vi "2-2.vi"() -> ()   [LabVIEW 2019, in "2.lvlib"]
uses:
  2.lvlib
  <vilib>/Utility/file.llb/Read Delimited Spreadsheet (string).vi
panel:
  out "XY Graph":cluster{i32[], i32[]}(graph)
  out "aim":i32
  out "depth x distance":i32
  out "distance":i32
  out "depth":i32
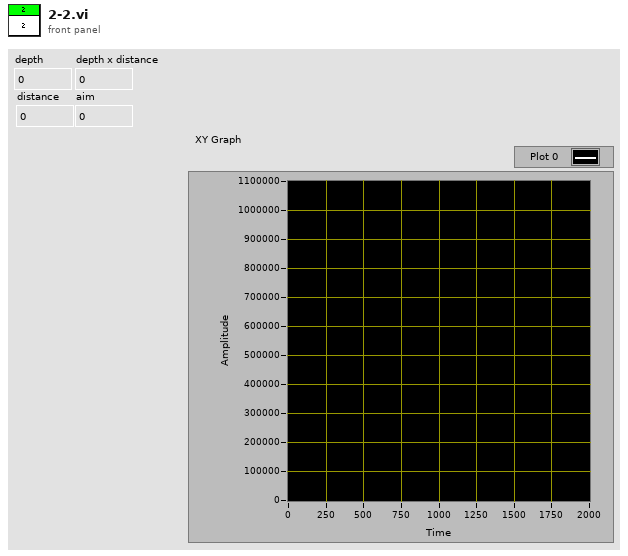
[diagram p1: front panel]
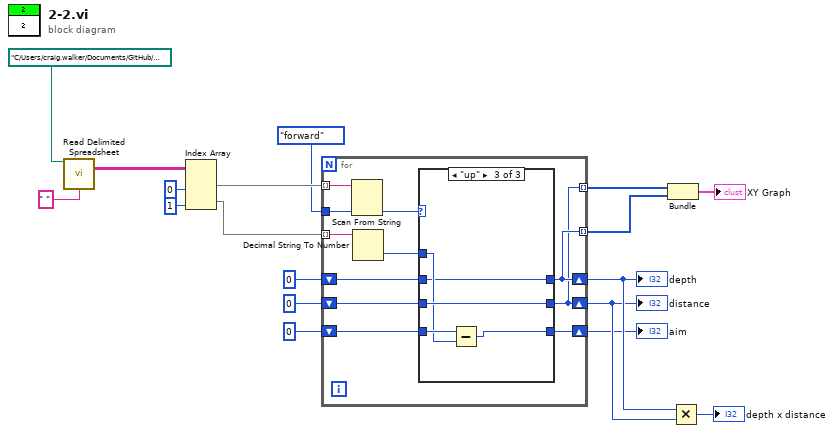
[diagram p0: block diagram]
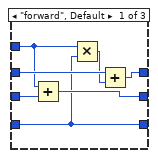
[diagram p2: hidden frame]
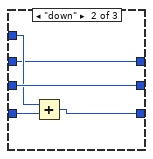
[diagram p3: hidden frame]
diagram:
  n1 = call-poly <vilib>:"Read Delimited Spreadsheet.vi"("file path (dialog if empty)"=path "C:/Users/craig.walker/Documents/GitHub/lv2019-Advent-of-Code-2021/2/input.txt", "delimiter (\\t)"=" " ("delimiter (\\t)")) -> ("all rows"=w1:string[][])  [unwired: 8 in, 5 out]
  n2 = Index Array(array=w1, index (col) #1=0 ("disabled index (col)"), index (col) #2=1 ("index (col)")) -> (element #1=w16:string[], element #2=w12:string[])  [unwired: 2 in]
  n3 = for {
    tunnel: w16 -> [w29] mode=indexing
    tunnel: enum16{"forward", "down", "up"}."forward" -> [w28]
    tunnel: w12 -> [w27] mode=indexing
    shift-right: [w20] -> w9
    shift-left: 0 -> [w25]
    shift-right: [w19] -> w8
    shift-left: 0 -> [w23]
    shift-right: [w21] -> w5
    shift-left: 0 -> [w22]
    tunnel: [w20] -> w3 mode=indexing
    tunnel: [w19] -> w2 mode=indexing
    n4 = Scan From String(input string=w29, default 1=w28) -> (output 1=w26:enum16{"forward", "down", "up"})  [unwired: 3 in, 3 out]
    n5 = Decimal String To Number(string=w27) -> (number=w24:i32)  [unwired: 2 in, 1 out]
    n6 = case shown="\"up\"" w26 {
      tunnel: w25 -> [w35 w37 w42]
      tunnel: w24 -> [w33 w39 w43]
      tunnel: [w31 w37 w42] -> w20
      tunnel: w23 -> [w36 w41 w46]
      tunnel: [w34 w41 w46] -> w19
      tunnel: w22 -> [w32 w40 w45]
      tunnel: [w32 w38 w44] -> w21
      frame "forward", Default {
        n7 = Add(x=w33, y=w36) -> (x+y=w34:i32)
        n8 = Multiply(x=w33, y=w32) -> (x*y=w30:i32)
        n9 = Add(x=w35, y=w30) -> (x+y=w31:i32)
      }
      frame "down" {
        n10 = Add(x=w39, y=w40) -> (x+y=w38:i32)
      }
      frame "up" {
        n11 = Subtract(x=w45, y=w43) -> (x-y=w44:i32)
      }
    }
  }
  "depth" <- w9
  "distance" <- w8
  "aim" <- w5
  n12 = Bundle(w2, w3) -> (→"XY Graph":cluster{i32[], i32[]})  [unwired: 1 in]
  n13 = Multiply(x=w9, y=w8) -> (x*y=→"depth x distance":i32)
